vi "Define.vi"(11 "Double Definition":T1) -> (3 "Double out":refnum<class "Double.lvclass">)   [LabVIEW 2020, in "Conditum.lvlib" / "Columns.lvlib" / "Double.lvclass"]
uses:
  Double.lvclass
  Type/Type.lvclass
  LabVIEW Type.ctl
  Conditum.lvlib
  Type/Definition.ctl
  Attributes.ctl
  Definition.ctl
  Double Definition.ctl
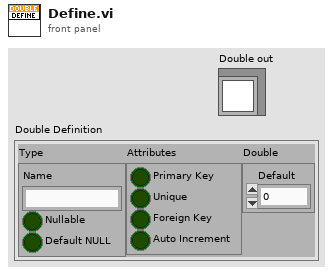
[diagram p1: front panel]
types:
  T1 = typedef "Conditum.lvlib/Columns.lvlib/Double.lvclass/Double Definition.ctl" = cluster{"Type":T2, "Attributes":T3, "Double":T4}
  T2 = typedef "Conditum.lvlib/Columns.lvlib/Type.lvclass/Definition.ctl" = cluster{"Name":string, "Nullable":bool, "Default NULL":bool}
  T3 = typedef "Conditum.lvlib/Attributes.ctl" = cluster{"Primary Key":bool, "Unique":bool, "Foreign Key":bool, "Auto Increment":bool}
  T4 = typedef "Conditum.lvlib/Columns.lvlib/Double.lvclass/Definition.ctl" = cluster{"Default":dbl}
  T5 = typedef "Conditum.lvlib/LabVIEW Type.ctl" = enum16{"None", "ID", "Boolean", "Integer", "Double", "Timestamp", "String", "Text", "Entity"}
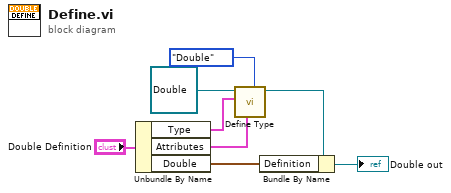
[diagram p0: block diagram]
diagram:
  n1 = Unbundle By Name("Double Definition") -> ("Type"=w6:T2, "Attributes"=w5:T3, "Double"=w4:T4)
  n2 = call "Define Type.vi"("Type"=LabVIEW_Type."Double", "Attributes"=w5, "Definition"=w6, "Type in"=refnum<class "Double.lvclass"> refnum ("Double in")) -> ("Type out"=w3:refnum<class "Double.lvclass">)  [unwired: 7 in]
  n3 = Bundle By Name(cluster=w3, "Definition"=w4) -> (→"Double out":refnum<class "Double.lvclass">)
